vi "MaxZ from Image array.vi"(7 "Image Type":T2 items=["Grayscale (U8)", "Grayscale (I16)", "Grayscale (SGL)", "Complex (CSG)", "RGB (U32)", "HSL (U32)", "RGB (U64)", "Grayscale (U16)"], 8 "error in (no error)":errorcluster, 11 "Array":T1[](array[plugin-control])) -> (0 "error out":errorcluster, 3 "Image 2":T1(plugin-control))   [LabVIEW 2017]
uses:
  <vilib>/vision/NI_Vision_Development_Module.lvlib
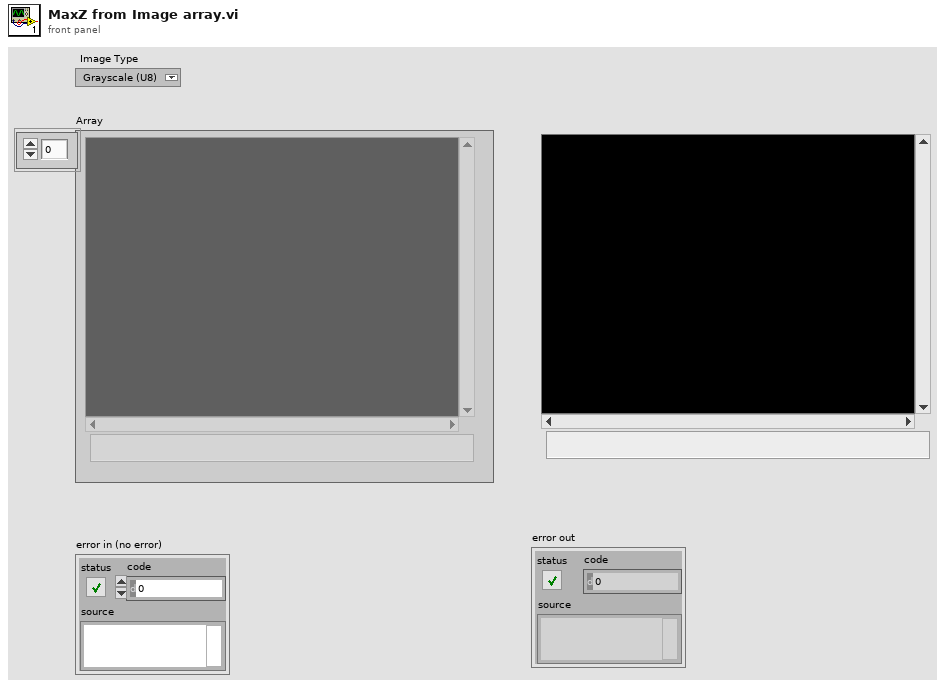
[diagram p1: front panel]
types:
  T1 = typedef "IMAQ Image.ctl" = refnum<image>
  T2 = typedef "Image Type" = u32
  T3 = enum32{"Average", "Min", "Max", "Clear  if < ", "Clear  if < or =", "Clear  if =", "Clear  if > or =", "Clear  if >"}
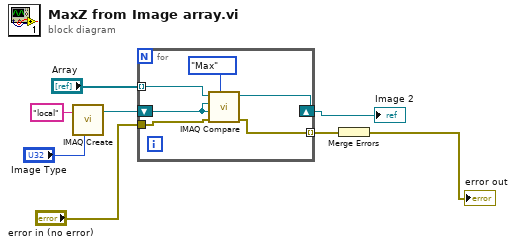
[diagram p0: block diagram]
diagram:
  n1 = call "IMAQ Create"("Image Name"="local", "Image Type"="Image Type") -> ("New Image"=w5:T1)  [unwired: 3 in, 1 out]
  n2 = for {
    tunnel: "Array" -> [w13] mode=indexing
    shift-right: [w12] -> w4
    shift-left: w5 -> [w11]
    tunnel: "error in (no error)" -> [w10]
    tunnel: [w9] -> w2 mode=indexing
    n3 = call "IMAQ Compare"("Operator"=T3."Max", "error in (no error)"=w10, "Image Src B"=w11, "Image Dst"=w11, "Image Src A"=w13) -> ("error out"=w9:errorcluster, "Image Dst Out"=w12:T1)  [unwired: 5 in]
  }
  "Image 2" <- w4
  n4 = Merge Errors(w2) -> (→"error out":errorcluster)
